vi "Configure Data Transition.vi"(7 "File Name ()":string, 8 "error in (no error)":errorcluster, 9 "Binary Block ()":string, 10 "Data Operation (0: Download Data)":i32(ring) items=["Download Data", "Store Data", "Upload Data"], 11 "VISA resource name":refnum<visa-resource-name>) -> (0 "error out":errorcluster, 3 "VISA resource name out":refnum<visa-resource-name>)   [LabVIEW 2013, in "Agilent 3446X Series.lvlib"]
doc: "Configures data transition settings."
uses:
  Agilent 3446X Series.lvlib
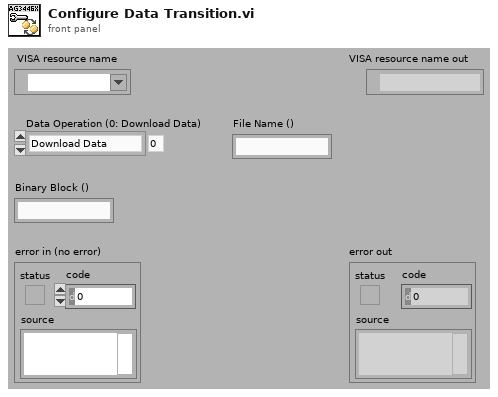
[diagram p1: front panel]
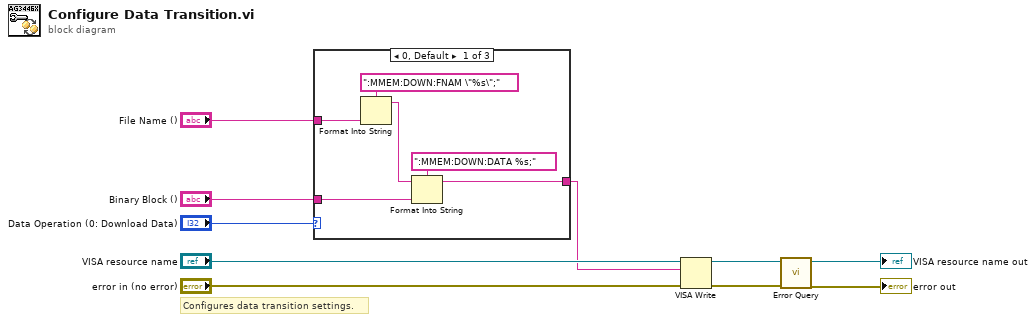
[diagram p0: block diagram]
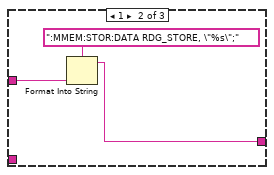
[diagram p2: hidden frame]
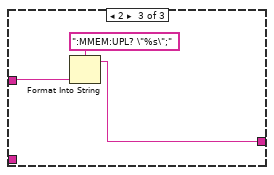
[diagram p3: hidden frame]
diagram:
  # "Configures data transition settings."
  n1 = case shown="0, Default" "Data Operation (0: Download Data)" {
    tunnel: "Binary Block ()" -> [w15 _ _]
    tunnel: [w14 w17 w20] -> w1
    tunnel: "File Name ()" -> [w12 w19 w21]
    frame 0, Default {
      n2 = Format Into String(format string=":MMEM:DOWN:FNAM \"%s\";", w12) -> (resulting string=w11:string)  [unwired: 2 in, 1 out]
      n3 = Format Into String(format string=":MMEM:DOWN:DATA %s;", initial string=w11, w15) -> (resulting string=w14:string)  [unwired: 1 in, 1 out]
    }
    frame 1 {
      n4 = Format Into String(format string=":MMEM:STOR:DATA RDG_STORE, \"%s\";", w19) -> (resulting string=w17:string)  [unwired: 2 in, 1 out]
    }
    frame 2 {
      n5 = Format Into String(format string=":MMEM:UPL? \"%s\";", w21) -> (resulting string=w20:string)  [unwired: 2 in, 1 out]
    }
  }
  n6 = VISA Write(VISA resource name="VISA resource name", write buffer=w1, error in (no error)="error in (no error)") -> (VISA resource name out=w8:refnum<visa-resource-name>, error out=w7:errorcluster)  [unwired: 1 out]
  n7 = call "Error Query.vi"("error in (no error)"=w7, "VISA resource name"=w8) -> ("error out"=→"error out":errorcluster, "VISA resource name out"=→"VISA resource name out":refnum<visa-resource-name>)  [unwired: 8 out]
